vi "Sistema de ventilación_V3.vi"() -> ()   [LabVIEW 2023]
uses:
  <vilib>/MakerHub/LINX/Public/Peripherals/Analog/Analog Read 1 Chan.vi
  <vilib>/MakerHub/LINX/Public/Peripherals/Digital/Digital Write 1 Chan.vi
  <vilib>/MakerHub/LINX/Public/Peripherals/Analog/Analog Read N Chans.vi
  <vilib>/MakerHub/LINX/Public/Peripherals/Digital/Digital Write N Chans.vi
  <vilib>/MakerHub/LINX/Private/Local IO/LinxAnalogRead.vi
  <vilib>/MakerHub/LINX/Public/Utilities/Check Channel.vi
  <vilib>/MakerHub/LINX/Private/Local IO/LinxDigitalWrite.vi
  <vilib>/MakerHub/LINX/Public/Utilities/Open Serial.vi
  <vilib>/MakerHub/LINX/Public/Sensors/Motion/Servo/Servo Open One Channel.vi
  <vilib>/MakerHub/LINX/Public/Peripherals/Analog/Analog Write 1 Chan.vi
  <vilib>/MakerHub/LINX/Private/Utilties/Generate Error.vi
  <vilib>/MakerHub/LINX/Public/Sensors/Temperature/TMP3x/TMP35.vi
  <vilib>/MakerHub/LINX/Public/Sensors/Motion/Servo/Servo Set Pulse Width One Channel.vi
  <vilib>/MakerHub/LINX/Public/Sensors/Motion/Servo/Servo Close One Channel.vi
  <vilib>/MakerHub/LINX/LMH-LINX.lvlib
  <vilib>/MakerHub/LINX/Public/Sensors/Temperature/TMP3x/TMP3x.lvlib
  <vilib>/MakerHub/LINX/Public/Sensors/Motion/Servo/Servo.lvlib
panel:
  in  "Temp":dbl(knob) scale=0.0..100.0
  in  "Aire":dbl(knob) scale=0.0..1000.0
  out "?":bool
  out "?":bool
  out "?":bool
  out "?":bool
  in  "?":bool
  out "Serevo Aire Angulo":string
  out "Serevo Temp Angulo":string
  in  "Serial Port":refnum<visa-resource-name>
  out "?":bool
  out "?":bool
  out "?":bool
  out "?":bool
  out "?":bool
  out "?":bool
  out "?":bool
  out "?":bool
  out "?":bool
  out "?":bool
  out "?":bool
  out "?":bool
  out "?":bool
  out "?":bool
  out "?":bool
  out "?":bool
  out "?":bool
  out "?":bool
  in  "?":bool
  out "Filtro de Calor":bool
  out "Filtro de Aire":bool
  out "Calidad del aire":dbl(knob) scale=0.0..1800.0
  out "Temperatura":dbl(slide) scale=0.0..60.0
  out "t [sec]":dbl
  out "Iteration No":i32
  in  "?":bool
  out "VI is running?":bool caption="ON/OFF"
  # "SISTEMA DE VENTILACIÓN DE DOBLE FLUJO"
  # "Entrada"
  # "Salida"
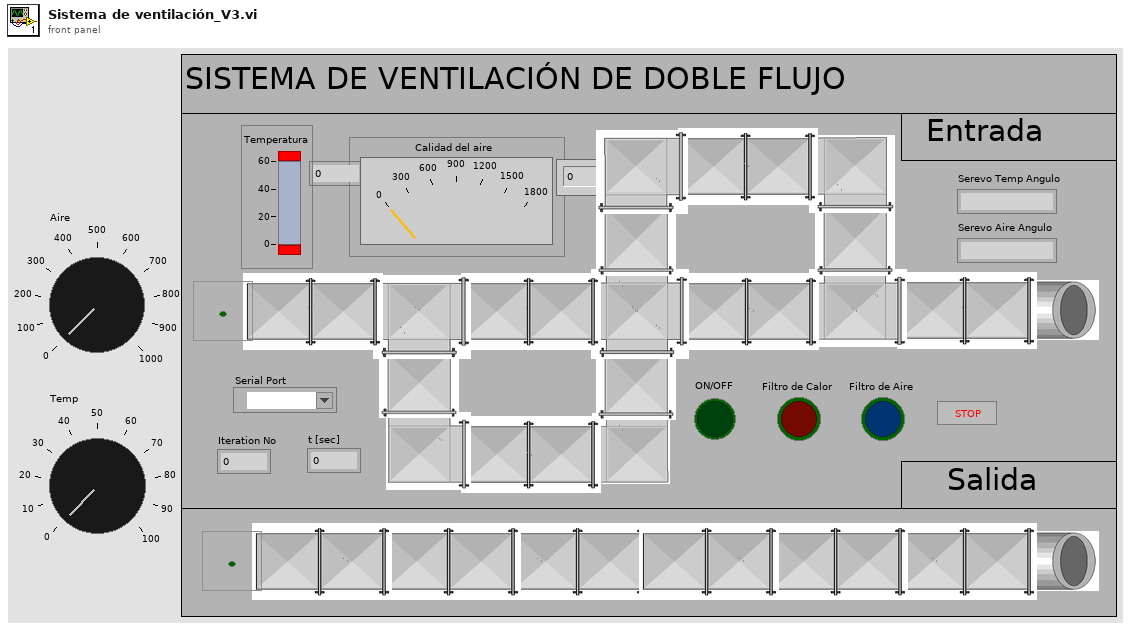
[diagram p1: front panel]
types:
  T1 = typedef "LMH-LINX.lvlib/LINX Ref.ctl" = cluster{"IO":T2, "Interface":T3, "LINX Device Config":T4}
  T2 = typedef "LMH-LINX.lvlib/Platform.ctl" = enum16{"Remote", "Local"}
  T3 = typedef "LMH-LINX.lvlib/Interface.ctl" = enum16{"Serial", "TCP"}
  T4 = typedef "LMH-LINX.lvlib/Device.lvlib/LINX Device Config.ctl" = cluster{"Interface":T3, "COM Port":refnum<visa-resource-name>, "TCP Configuration":T5, "Device Family":u8, "Device ID":u8, "Device Name":string, "TCP Ref":refnum<k5>, "Channels":T6}
  T5 = typedef "LMH-LINX.lvlib/Device.lvlib/TCP Config.ctl" = cluster{"IP Address":string, "Port":u16}
  T6 = typedef "LMH-LINX.lvlib/Channels.ctl" = cluster{"DI":u8[], "DO":u8[], "AI":u8[], "AO":u8[], "PWM":u8[], "QE":u8[], "UART":u8[], "I2C 2":u8[], "SPI":u8[], "CAN":u8[], "Servo":u8[], "AI Ref (V)":dbl, "AI Resolution (Bits)":u8, "AO Ref (V)":dbl, "AO Resolution (Bits)":u8}
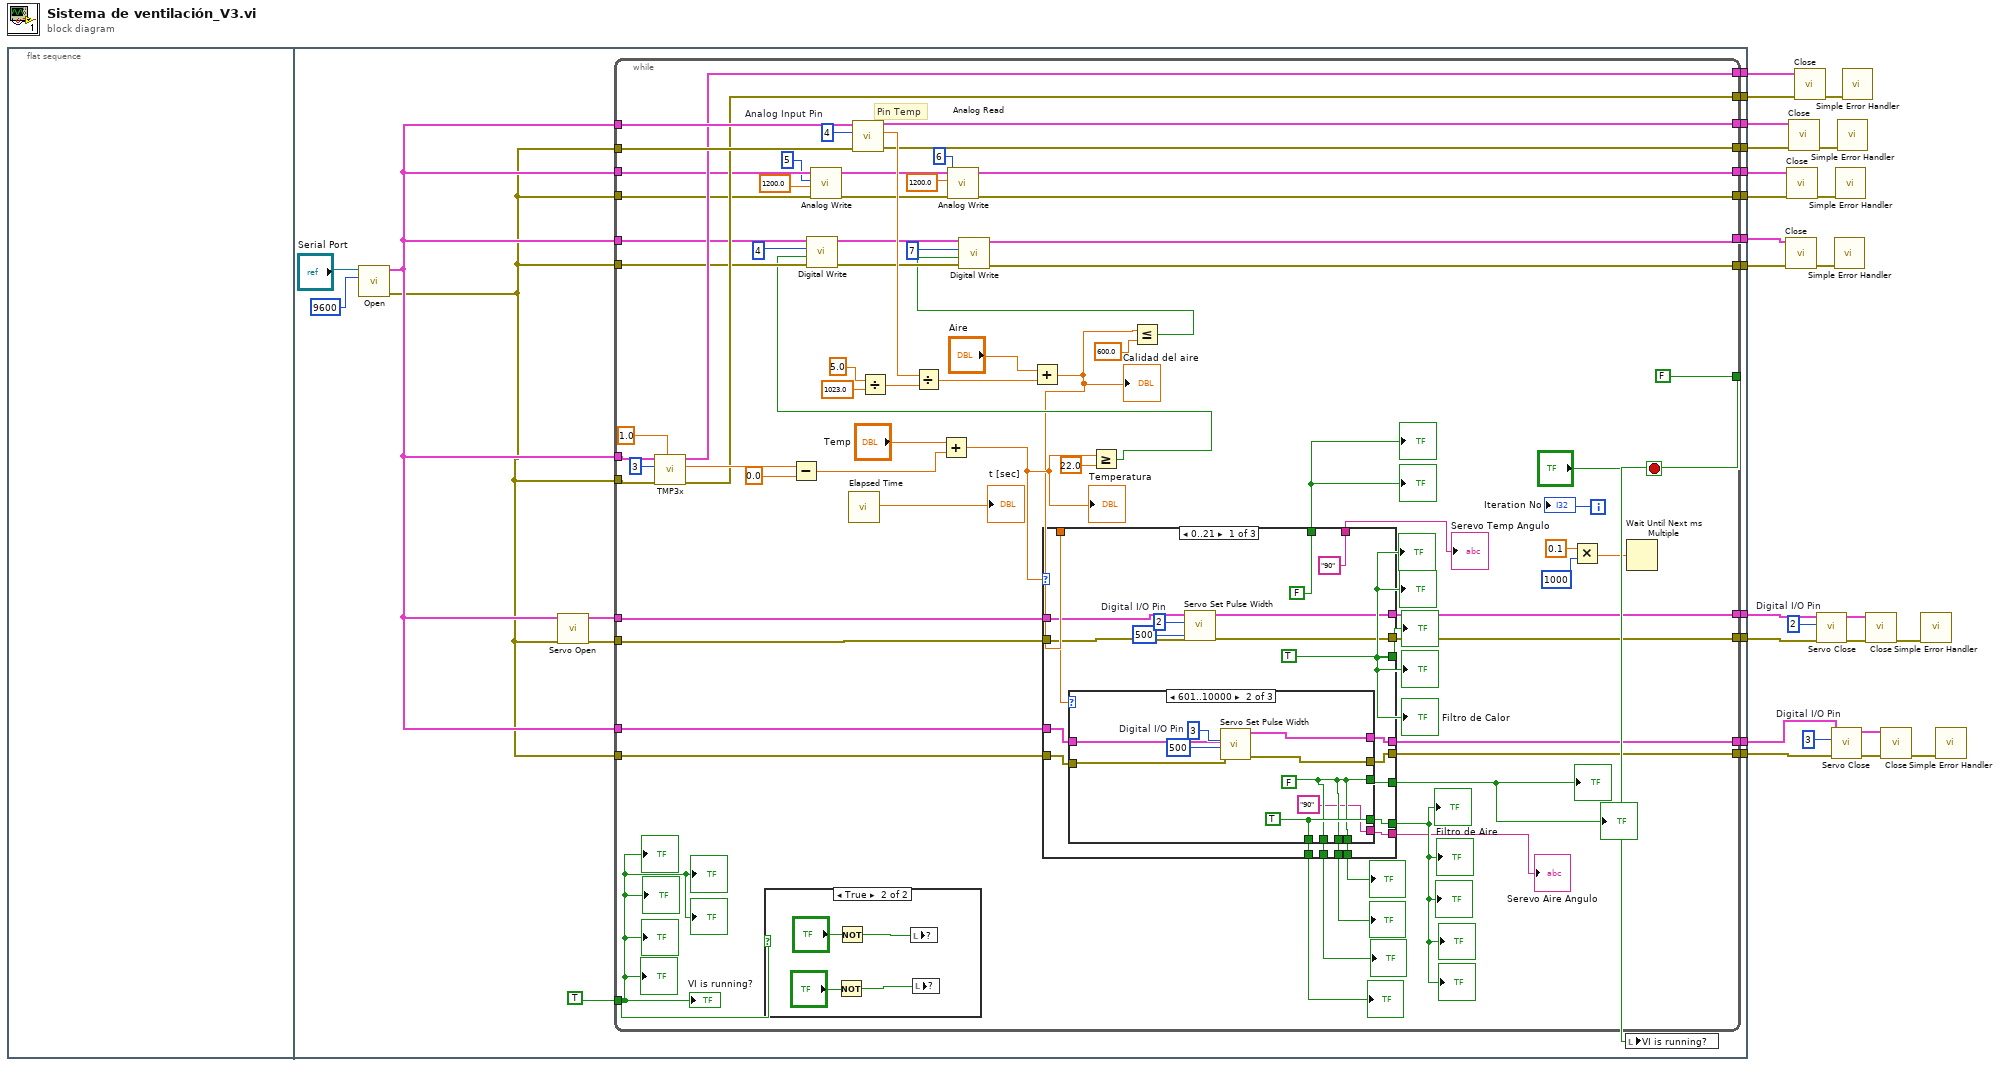
[diagram p0: block diagram]
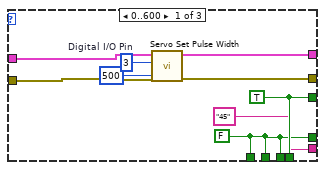
[diagram p2: hidden frame]
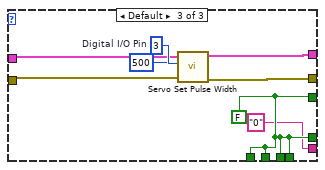
[diagram p3: hidden frame]
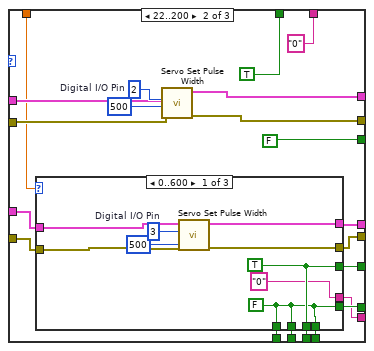
[diagram p4: hidden frame]
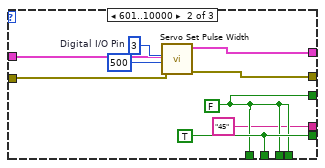
[diagram p5: hidden frame]
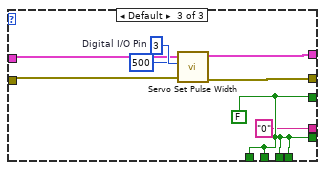
[diagram p6: hidden frame]
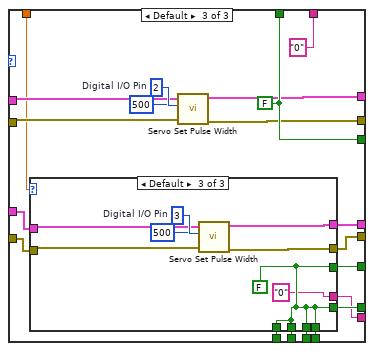
[diagram p7: hidden frame]
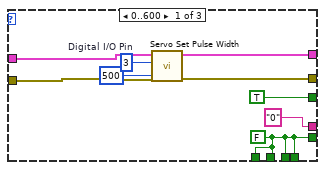
[diagram p8: hidden frame]
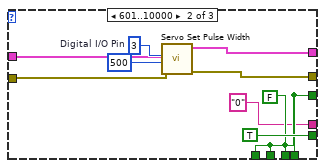
[diagram p9: hidden frame]
diagram:
  w6 = 3  # Digital I/O Pin
  w12 = 2  # Digital I/O Pin
  n1 = flat-sequence {
    tunnel: [w41] -> w24
    tunnel: [w39] -> w22
    tunnel: [w38] -> w20
    tunnel: [w37] -> w19
    tunnel: [w36] -> w17
    tunnel: [w35] -> w16
    tunnel: [w34] -> w14
    tunnel: [w33] -> w13
    tunnel: [w30] -> w8
    tunnel: [w29] -> w7
    tunnel: [w26] -> w2
    tunnel: [w25] -> w1
    frame #0 {
    }
    frame #1 {
      n2 = call-poly <vilib>:"Open.vi"("Baud Rate Override"=u32 9600, "Serial Port"="Serial Port") -> ("Error Out"=w27:errorcluster, "LINX Resource"=w28:T1)  [unwired: 7 in, 1 out]
      n3 = call-poly <vilib>:"Servo Open.vi"("Error In"=w27, "LINX Resource"=w28) -> ("Error Out"=w31:errorcluster, "LINX Resource"=w32:T1)  [unwired: 8 in]
      n4 = while {
        tunnel: [FALSE] -> w43
        tunnel: TRUE -> [w81]
        tunnel: w28 -> [w108]
        tunnel: [w94] -> w41
        tunnel: w27 -> [w106]
        tunnel: w28 -> [w103]
        tunnel: [w95] -> w39
        tunnel: w27 -> [w98]
        tunnel: [w93] -> w38
        tunnel: [w92] -> w37
        tunnel: w27 -> [w91]
        tunnel: w28 -> [w90]
        tunnel: [w83] -> w36
        tunnel: [w82] -> w35
        tunnel: w27 -> [w80]
        tunnel: w28 -> [w79]
        tunnel: [w74] -> w34
        tunnel: [w73] -> w33
        tunnel: w32 -> [w70]
        tunnel: w31 -> [w69]
        tunnel: [w68] -> w30
        tunnel: [w67] -> w29
        tunnel: w28 -> [w58]
        tunnel: w27 -> [w57]
        tunnel: [w56] -> w26
        tunnel: [w55] -> w25
        i -> [w110]
        stop <- "?" stop-if-true
        w97 = 4  # Analog Input Pin
        # "Pin Temp"
        n5 = call-poly <vilib>:"TMP3x.vi"("Analog Ref Override"=1.0, "Error In"=w106, "Analog Channel"=3, "LINX Resource"=w108) -> ("Error Out"=w95:errorcluster, "Temp C"=w104:dbl, "LINX Resource"=w94:T1)  [unwired: 5 in]
        n6 = case shown="True" w81 {
          frame False {
          }
          frame True {
            n7 = Not(x="?") -> (.not. x?=w256:bool)
            n8 = Not(x="?") -> (.not. x?=w258:bool)
            n9 = local write item#8(w258) -> ()
            n10 = local write item#30(w256) -> ()
          }
        }
        n11 = Subtract(x=w104, y=0.0) -> (x-y=w63:dbl)
        n12 = call-poly <vilib>:"Analog Write.vi"("Error In"=w91, "AO Value"=1200.0, "AO Channel"=5, "LINX Resource"=w90) -> ("Error Out"=w84:errorcluster, "LINX Resource"=w85:T1)  [unwired: 6 in]
        n13 = call "Elapsed Time"() -> ("Elapsed Time (s)"=→"t [sec]":dbl)  [unwired: 12 in, 7 out]
        n14 = call-poly <vilib>:"Analog Read.vi"("Error In"=w98, "Analog Channel"=w97, "LINX Resource"=w103) -> ("Error Out"=w92:errorcluster, "Voltage"=w100:dbl, "LINX Resource"=w93:T1)  [unwired: 5 in, 1 out]
        n15 = Divide(x=5.0, y=1023.0) -> (x/y=w99:dbl)
        n16 = Divide(x=w100, y=w99) -> (x/y=w65:dbl)
        n17 = Add(x="Temp", y=w63) -> (x+y=w61:dbl)
        "Temperatura" <- w61
        n18 = call-poly <vilib>:"Analog Write.vi"("Error In"=w84, "AO Value"=1200.0, "AO Channel"=6, "LINX Resource"=w85) -> ("Error Out"=w83:errorcluster, "LINX Resource"=w82:T1)  [unwired: 6 in]
        n19 = Add(x="Aire", y=w65) -> (x+y=w54:dbl)
        "Calidad del aire" <- w54
        n20 = case shown="0..21" w61 {
          tunnel: w70 -> [w134 w181 w226]
          tunnel: w69 -> [w133 w180 w225]
          tunnel: [w132 w179 w223] -> w68
          tunnel: [w131 w178 w224] -> w67
          tunnel: [TRUE FALSE w229] -> w60
          tunnel: [FALSE TRUE w229] -> w59
          tunnel: w58 -> [w125 w170 w222]
          tunnel: w57 -> [w124 w169 w221]
          tunnel: [w122 w171 w220] -> w56
          tunnel: [w123 w172 w219] -> w55
          tunnel: w54 -> [w126 w173 w218]
          tunnel: [w128 w175 w217] -> w52
          tunnel: [w127 w174 w216] -> w51
          tunnel: [w121 w168 w212] -> w50
          tunnel: [w118 w167 w213] -> w49
          tunnel: [w119 w166 w214] -> w48
          tunnel: [w120 w165 w215] -> w47
          tunnel: ["90" ("Serevo Temp Angulo") "0" ("Serevo Temp Angulo") "0" ("Serevo Temp Angulo")] -> w46
          tunnel: [w116 w163 w210] -> w45
          frame 0..21 {
            w136 = 2  # Digital I/O Pin
            n21 = case shown="601..10000" w126 {
              tunnel: w125 -> [w143 w152 w160]
              tunnel: w124 -> [w142 w151 w159]
              tunnel: [w141 w150 w157] -> w123
              tunnel: [w140 w149 w158] -> w122
              tunnel: [w139 w147 w156] -> w128
              tunnel: [w138 w148 w156] -> w127
              tunnel: [w139 w147 w156] -> w121
              tunnel: [w138 w148 w156] -> w120
              tunnel: [w138 w147 w156] -> w119
              tunnel: [w138 w147 w156] -> w118
              tunnel: ["45" ("Serevo Aire Angulo") "90" ("Serevo Aire Angulo") "0" ("Serevo Aire Angulo")] -> w116
              frame 0..600 {
                w138 = FALSE
                w139 = TRUE
                w145 = 3  # Digital I/O Pin
                n22 = call-poly <vilib>:"Servo Set Pulse Width.vi"("Error In"=w142, "Pulse Width (uS)"=u16 500, "Servo Channel"=w145, "LINX Resource"=w143) -> ("Error Out"=w140:errorcluster, "LINX Resource"=w141:T1)  [unwired: 6 in]
              }
              frame 601..10000 {
                w147 = FALSE
                w148 = TRUE
                w154 = 3  # Digital I/O Pin
                n23 = call-poly <vilib>:"Servo Set Pulse Width.vi"("Error In"=w151, "Pulse Width (uS)"=u16 500, "Servo Channel"=w154, "LINX Resource"=w152) -> ("Error Out"=w149:errorcluster, "LINX Resource"=w150:T1)  [unwired: 6 in]
              }
              frame Default {
                w162 = 3  # Digital I/O Pin
                w156 = FALSE
                n24 = call-poly <vilib>:"Servo Set Pulse Width.vi"("Error In"=w159, "Pulse Width (uS)"=u16 500, "Servo Channel"=w162, "LINX Resource"=w160) -> ("Error Out"=w158:errorcluster, "LINX Resource"=w157:T1)  [unwired: 6 in]
              }
            }
            n25 = call-poly <vilib>:"Servo Set Pulse Width.vi"("Error In"=w133, "Pulse Width (uS)"=u16 500, "Servo Channel"=w136, "LINX Resource"=w134) -> ("Error Out"=w131:errorcluster, "LINX Resource"=w132:T1)  [unwired: 6 in]
          }
          frame 22..200 {
            w183 = 2  # Digital I/O Pin
            n26 = case shown="0..600" w173 {
              tunnel: w170 -> [w190 w199 w207]
              tunnel: w169 -> [w189 w198 w206]
              tunnel: [w188 w197 w204] -> w172
              tunnel: [w187 w196 w205] -> w171
              tunnel: [w186 w194 w203] -> w175
              tunnel: [w185 w195 w203] -> w174
              tunnel: [w185 w194 w203] -> w168
              tunnel: [w186 w194 w203] -> w167
              tunnel: [w185 w195 w203] -> w166
              tunnel: [w185 w194 w203] -> w165
              tunnel: ["0" ("Serevo Aire Angulo") "45" ("Serevo Aire Angulo") "0" ("Serevo Aire Angulo")] -> w163
              frame 0..600 {
                w185 = FALSE
                w186 = TRUE
                w192 = 3  # Digital I/O Pin
                n27 = call-poly <vilib>:"Servo Set Pulse Width.vi"("Error In"=w189, "Pulse Width (uS)"=u16 500, "Servo Channel"=w192, "LINX Resource"=w190) -> ("Error Out"=w187:errorcluster, "LINX Resource"=w188:T1)  [unwired: 6 in]
              }
              frame 601..10000 {
                w194 = FALSE
                w195 = TRUE
                w201 = 3  # Digital I/O Pin
                n28 = call-poly <vilib>:"Servo Set Pulse Width.vi"("Error In"=w198, "Pulse Width (uS)"=u16 500, "Servo Channel"=w201, "LINX Resource"=w199) -> ("Error Out"=w196:errorcluster, "LINX Resource"=w197:T1)  [unwired: 6 in]
              }
              frame Default {
                w209 = 3  # Digital I/O Pin
                w203 = FALSE
                n29 = call-poly <vilib>:"Servo Set Pulse Width.vi"("Error In"=w206, "Pulse Width (uS)"=u16 500, "Servo Channel"=w209, "LINX Resource"=w207) -> ("Error Out"=w205:errorcluster, "LINX Resource"=w204:T1)  [unwired: 6 in]
              }
            }
            n30 = call-poly <vilib>:"Servo Set Pulse Width.vi"("Error In"=w180, "Pulse Width (uS)"=u16 500, "Servo Channel"=w183, "LINX Resource"=w181) -> ("Error Out"=w178:errorcluster, "LINX Resource"=w179:T1)  [unwired: 6 in]
          }
          frame Default {
            w228 = 2  # Digital I/O Pin
            w229 = FALSE
            n31 = case shown="Default" w218 {
              tunnel: w222 -> [w236 w245 w253]
              tunnel: w221 -> [w235 w244 w252]
              tunnel: [w234 w243 w250] -> w219
              tunnel: [w233 w242 w251] -> w220
              tunnel: [TRUE w240 w249] -> w217
              tunnel: [w231 TRUE w249] -> w216
              tunnel: [w231 w240 w249] -> w215
              tunnel: [w231 w240 w249] -> w214
              tunnel: [w231 w240 w249] -> w213
              tunnel: [w231 w240 w249] -> w212
              tunnel: ["0" ("Serevo Aire Angulo") "0" ("Serevo Aire Angulo") "0" ("Serevo Aire Angulo")] -> w210
              frame 0..600 {
                w231 = FALSE
                w238 = 3  # Digital I/O Pin
                n32 = call-poly <vilib>:"Servo Set Pulse Width.vi"("Error In"=w235, "Pulse Width (uS)"=u16 500, "Servo Channel"=w238, "LINX Resource"=w236) -> ("Error Out"=w233:errorcluster, "LINX Resource"=w234:T1)  [unwired: 6 in]
              }
              frame 601..10000 {
                w240 = FALSE
                w247 = 3  # Digital I/O Pin
                n33 = call-poly <vilib>:"Servo Set Pulse Width.vi"("Error In"=w244, "Pulse Width (uS)"=u16 500, "Servo Channel"=w247, "LINX Resource"=w245) -> ("Error Out"=w242:errorcluster, "LINX Resource"=w243:T1)  [unwired: 6 in]
              }
              frame Default {
                w255 = 3  # Digital I/O Pin
                w249 = FALSE
                n34 = call-poly <vilib>:"Servo Set Pulse Width.vi"("Error In"=w252, "Pulse Width (uS)"=u16 500, "Servo Channel"=w255, "LINX Resource"=w253) -> ("Error Out"=w251:errorcluster, "LINX Resource"=w250:T1)  [unwired: 6 in]
              }
            }
            n35 = call-poly <vilib>:"Servo Set Pulse Width.vi"("Error In"=w225, "Pulse Width (uS)"=u16 500, "Servo Channel"=w228, "LINX Resource"=w226) -> ("Error Out"=w224:errorcluster, "LINX Resource"=w223:T1)  [unwired: 6 in]
          }
        }
        "?" <- w48
        "?" <- w49
        "?" <- w47
        "?" <- w50
        "Serevo Temp Angulo" <- w46
        "Serevo Aire Angulo" <- w45
        "?" <- w60
        "?" <- w60
        "?" <- w60
        "?" <- w60
        "Filtro de Calor" <- w60
        "?" <- w59
        "?" <- w59
        "Filtro de Aire" <- w51
        "?" <- w51
        "?" <- w51
        "?" <- w51
        "?" <- w51
        "?" <- w52
        "?" <- w52
        n36 = Greater Or Equal?(x=w61, y=22.0) -> (x >= y?=w62:bool)
        n37 = call-poly <vilib>:"Digital Write.vi"("Error In"=w80, "Output Value"=w62, "DO Channel"=4, "LINX Resource"=w79) -> ("Error Out"=w75:errorcluster, "LINX Resource"=w76:T1)  [unwired: 6 in]
        n38 = Less Or Equal?(x=w54, y=600.0) -> (x <= y?=w53:bool)
        n39 = call-poly <vilib>:"Digital Write.vi"("Error In"=w75, "Output Value"=w53, "DO Channel"=7, "LINX Resource"=w76) -> ("Error Out"=w73:errorcluster, "LINX Resource"=w74:T1)  [unwired: 6 in]
        n40 = Multiply(x=0.1, y=1000) -> (x*y=w113:dbl)
        n41 = Wait Until Next ms Multiple(millisecond multiple=w113) -> ()  [unwired: 1 out]
        "VI is running?" <- w81
        "Iteration No" <- w110
        "?" <- w81
        "?" <- w81
        "?" <- w81
        "?" <- w81
        "?" <- w81
        "?" <- w81
      }
      n42 = local write "VI is running?"(w43) -> ()
    }
  }
  n43 = call <vilib>:"Close.vi"("Error In"=w13, "LINX Resource"=w14) -> ("Error Out"=w15:errorcluster)  [unwired: 9 in]
  n44 = call <vilib>:"Close.vi"("Error In"=w17, "LINX Resource"=w16) -> ("Error Out"=w18:errorcluster)  [unwired: 9 in]
  n45 = call <vilib>:"Close.vi"("Error In"=w19, "LINX Resource"=w20) -> ("Error Out"=w21:errorcluster)  [unwired: 9 in]
  n46 = call <vilib>:"Close.vi"("Error In"=w22, "LINX Resource"=w24) -> ("Error Out"=w23:errorcluster)  [unwired: 9 in]
  n47 = call-poly <vilib>:"Servo Close.vi"("Error In"=w7, "Servo Channel"=w12, "LINX Resource"=w8) -> ("Error Out"=w10:errorcluster, "LINX Resource"=w11:T1)  [unwired: 7 in]
  n48 = call-poly <vilib>:"Servo Close.vi"("Error In"=w2, "Servo Channel"=w6, "LINX Resource"=w1) -> ("Error Out"=w4:errorcluster, "LINX Resource"=w5:T1)  [unwired: 7 in]
  n49 = call <vilib>:"Simple Error Handler.vi"("error in (no error)"=w15) -> ()  [unwired: 4 in, 5 out]
  n50 = call <vilib>:"Simple Error Handler.vi"("error in (no error)"=w18) -> ()  [unwired: 4 in, 5 out]
  n51 = call <vilib>:"Simple Error Handler.vi"("error in (no error)"=w21) -> ()  [unwired: 4 in, 5 out]
  n52 = call <vilib>:"Simple Error Handler.vi"("error in (no error)"=w23) -> ()  [unwired: 4 in, 5 out]
  n53 = call <vilib>:"Close.vi"("Error In"=w10, "LINX Resource"=w11) -> ("Error Out"=w9:errorcluster)  [unwired: 9 in]
  n54 = call <vilib>:"Close.vi"("Error In"=w4, "LINX Resource"=w5) -> ("Error Out"=w3:errorcluster)  [unwired: 9 in]
  n55 = call <vilib>:"Simple Error Handler.vi"("error in (no error)"=w9) -> ()  [unwired: 4 in, 5 out]
  n56 = call <vilib>:"Simple Error Handler.vi"("error in (no error)"=w3) -> ()  [unwired: 4 in, 5 out]
